vi "PW3337_Open232.vi"(8 "error in (no error)":errorcluster, 10 "baud rate (9600)":u32=9600, 11 "VISA resource name":refnum<visa-resource-name>) -> (0 "error out":errorcluster, 3 "status":bool)   [LabVIEW 2017]
uses:
  <vilib>/Instr/_visa.llb/VISA Configure Serial Port (Instr).vi
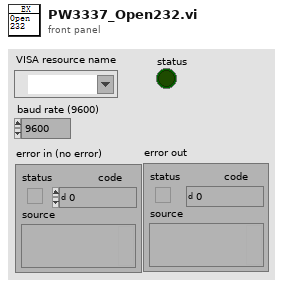
[diagram p1: front panel]
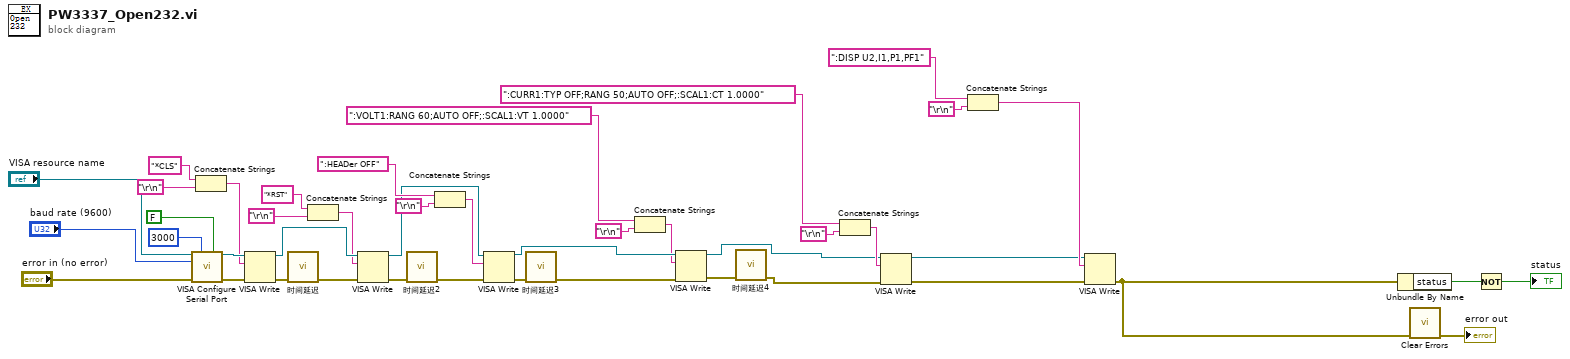
[diagram p0: block diagram]
diagram:
  n1 = call-poly "VISA Configure Serial Port"("VISA resource name"="VISA resource name", "timeout (10sec)"=u32 3000, "Enable Termination\nChar (T)"=FALSE ("Enable Termination\nChar (T)"), "baud rate (9600)"="baud rate (9600)", "error in (no error)"="error in (no error)") -> ("VISA resource name out"=w34:refnum<visa-resource-name>, "error out"=w40:errorcluster)  [unwired: 9 in]
  n2 = Concatenate Strings("*CLS" ("写入缓冲区"), "\r\n") -> (w32:string)
  n3 = VISA Write(VISA resource name=w34, write buffer=w32, error in (no error)=w40) -> (VISA resource name out=w28:refnum<visa-resource-name>, error out=w21:errorcluster)  [unwired: 1 out]
  n4 = call "时间延迟"("error in (no error)"=w21) -> ("error out"=w20:errorcluster)  [unwired: 10 in]
  n5 = Concatenate Strings("*RST" ("写入缓冲区"), "\r\n") -> (w27:string)
  n6 = VISA Write(VISA resource name=w28, write buffer=w27, error in (no error)=w20) -> (VISA resource name out=w24:refnum<visa-resource-name>, error out=w22:errorcluster)  [unwired: 1 out]
  n7 = call "时间延迟2"("error in (no error)"=w22) -> ("error out"=w19:errorcluster)  [unwired: 10 in]
  n8 = Concatenate Strings(":HEADer OFF", "\r\n") -> (w23:string)
  n9 = VISA Write(VISA resource name=w24, write buffer=w23, error in (no error)=w19) -> (VISA resource name out=w16:refnum<visa-resource-name>, error out=w18:errorcluster)  [unwired: 1 out]
  n10 = call "时间延迟3"("error in (no error)"=w18) -> ("error out"=w17:errorcluster)  [unwired: 10 in]
  n11 = Concatenate Strings(":VOLT1:RANG 60;AUTO OFF;:SCAL1:VT 1.0000" ("concatenated string"), "\r\n") -> (w14:string)
  n12 = VISA Write(VISA resource name=w16, write buffer=w14, error in (no error)=w17) -> (VISA resource name out=w8:refnum<visa-resource-name>, error out=w11:errorcluster)  [unwired: 1 out]
  n13 = call "时间延迟4"("error in (no error)"=w11) -> ("error out"=w10:errorcluster)  [unwired: 10 in]
  n14 = Concatenate Strings(":CURR1:TYP OFF;RANG 50;AUTO OFF;:SCAL1:CT 1.0000" ("concatenated string"), "\r\n") -> (w13:string)
  n15 = VISA Write(VISA resource name=w8, write buffer=w13, error in (no error)=w10) -> (VISA resource name out=w2:refnum<visa-resource-name>, error out=w4:errorcluster)  [unwired: 1 out]
  n16 = Concatenate Strings(":DISP U2,I1,P1,PF1" ("string"), "\r\n") -> (w5:string)
  n17 = VISA Write(VISA resource name=w2, write buffer=w5, error in (no error)=w4) -> (error out=w3:errorcluster)  [unwired: 2 out]
  n18 = Unbundle By Name(w3) -> ("status"=w38:bool)
  n19 = call <vilib>:"Clear Errors.vi"("error in (no error)"=w3) -> ("error out"=→"error out":errorcluster)  [unwired: 5 in, 1 out]
  n20 = Not(x=w38) -> (.not. x?=→"status":bool)
